vi "TDMS read for square (2).vi"() -> ()   [LabVIEW 2018]
uses:
  <vilib>/Analysis/Matrix/Numeric/Conversions/Array To Matrix - RA2.vi
  <vilib>/Analysis/Matrix/Numeric/Conversions/Matrix To Array - RM.vi
  <vilib>/Analysis/Matrix/NI_Matrix.lvlib
panel:
  out "result string":string
  out "string":string
  out "4":i32
  out "3":i32
  out "2":i32
  out "1":i32
  out "square X axis":dbl[][](graph)
  out "square Y axis":dbl[][](graph)
  in  "Scale:Multiplier":dbl=0.1
  in  "X Scale:Offset":dbl
  in  "Y Scale:Offset":dbl
  out "String":string
  in  "End Vector X":dbl
  in  "Start Vector X":dbl
  in  "End Vector Y":dbl
  in  "Start Vector Y":dbl
  out "Intensity Graph":dbl[][](graph)
  out "original X axis":dbl[][](graph)
  out "original Y axis":dbl[][](graph)
  in  "file path":path
  in  "OK Button":bool
  # "left side looking direction"
  # "right side looking direction"
  # "right side looking direction"
  # "left side looking direction"
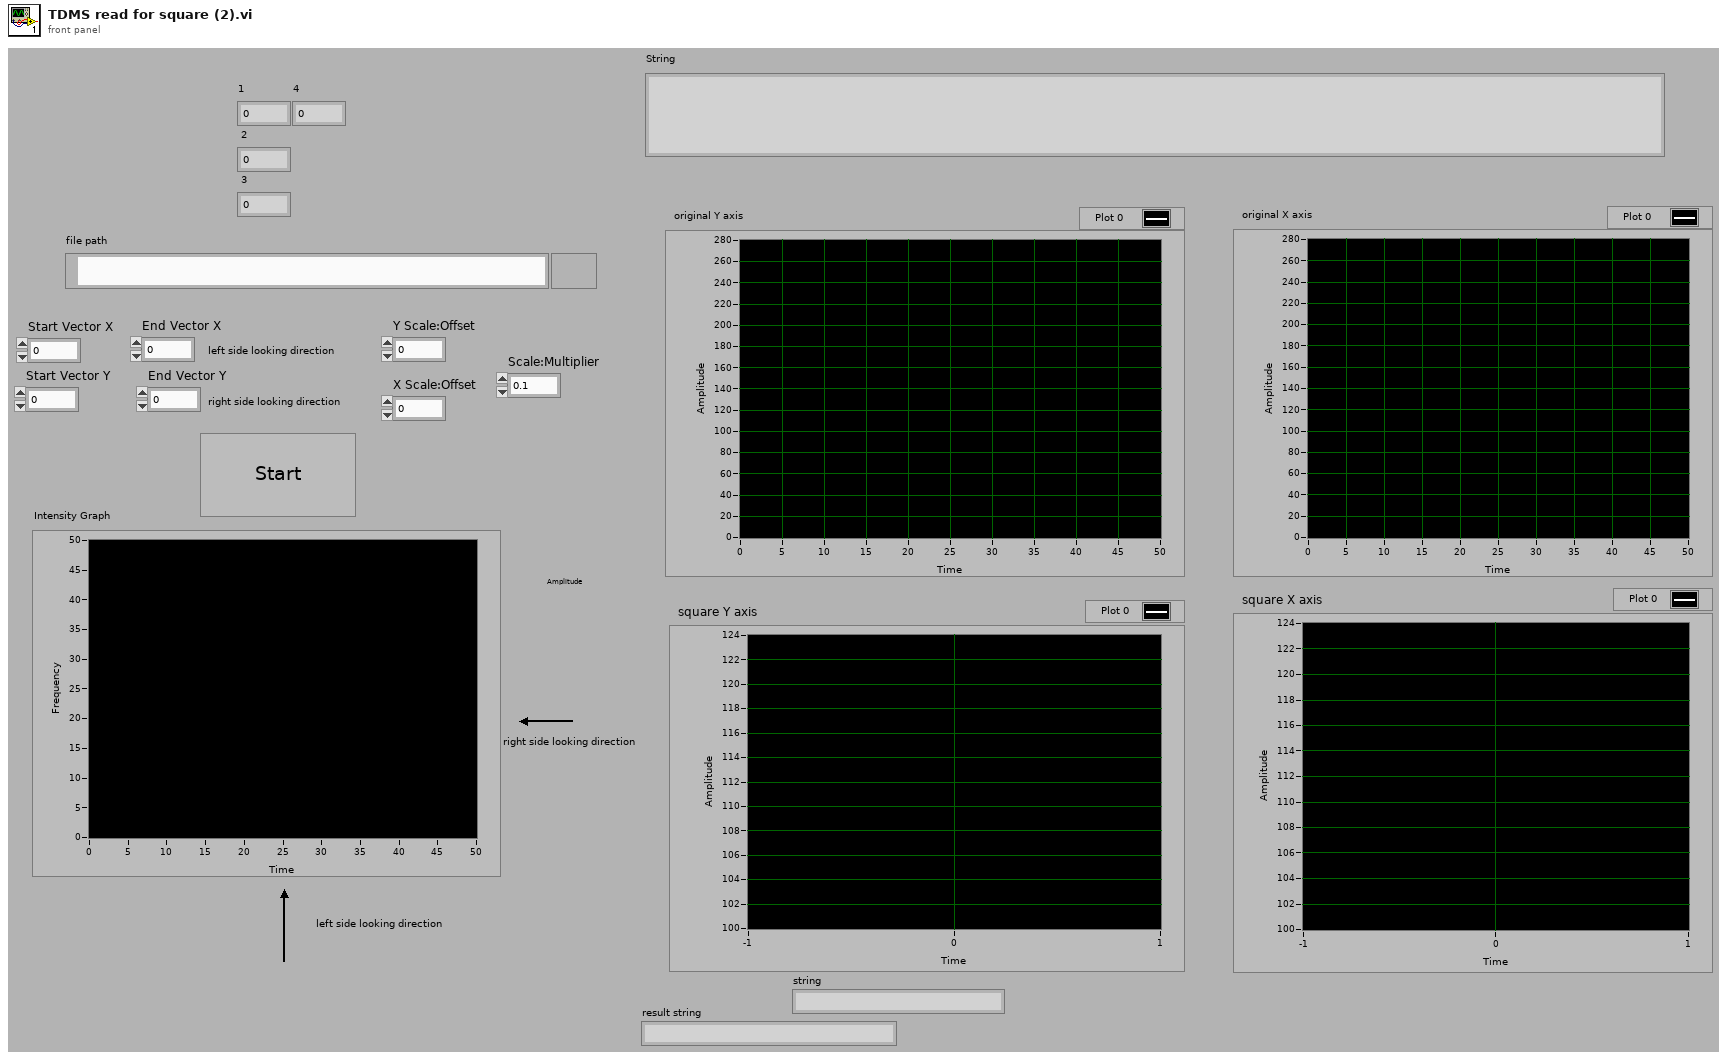
[diagram p1: front panel]
types:
  T1 = enum16{"open", "replace", "create", "open or create", "replace or create", "replace or create with confirmation"}
  T2 = enum16{"open", "open or create", "create or replace", "create", "open (read-only)"}
  T3 = typedef "NI_Matrix.lvlib/RealMatrix.ctl" = dbl[][]
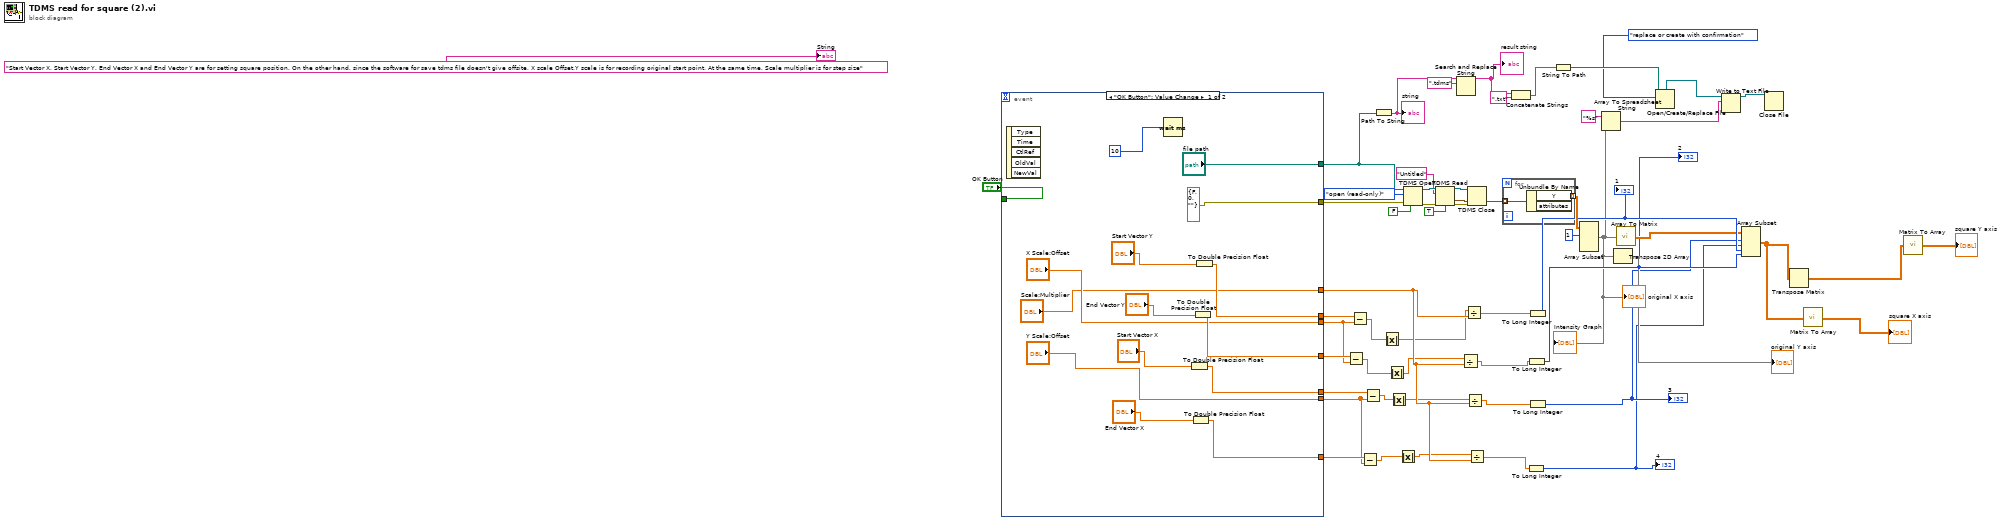
[diagram p0: block diagram]
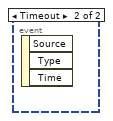
[diagram p2: hidden frame]
diagram:
  n1 = event shown="[0] \"OK Button\": Value Change" {
    selector: _ -> [_ _]
    dyn-events: _ -> [_ _]
    timeout: _ -> [_ _]
    tunnel: "OK Button" -> [_ _]
    tunnel: ["file path" _] -> w13
    tunnel: [errorcluster {"status"=FALSE, "code"=0, "source"=""} ("error constant") _] -> w46
    tunnel: [w66 _] -> w42
    tunnel: [w64 _] -> w41
    tunnel: [w61 _] -> w40
    tunnel: [w60 _] -> w39
    tunnel: ["X Scale:Offset" _] -> w38
    tunnel: ["Y Scale:Offset" _] -> w37
    tunnel: ["Scale:Multiplier" _] -> w36
    event "OK Button": Value Change {
      n2 = event-data() -> ()  [unwired: 1 in, 5 out]
      n3 = Wait (ms)(milliseconds to wait=u32 10) -> ()  [unwired: 1 out]
      n4 = To Double Precision Float(number="Start Vector X") -> (double precision float=w66:dbl)
      n5 = To Double Precision Float(number="End Vector X") -> (double precision float=w64:dbl)
      n6 = To Double Precision Float(number="End Vector Y") -> (double precision float=w60:dbl)
      n7 = To Double Precision Float(number="Start Vector Y") -> (double precision float=w61:dbl)
    }
    event Timeout {
      n8 = event-data() -> ()  [unwired: 1 in, 3 out]
    }
  }
  n9 = Subtract(x=w39, y=w38) -> (x-y=w29:dbl)
  n10 = Subtract(x=w40, y=w38) -> (x-y=w35:dbl)
  n11 = Subtract(x=w41, y=w37) -> (x-y=w33:dbl)
  n12 = Subtract(x=w42, y=w37) -> (x-y=w31:dbl)
  n13 = Path To String(path=w13) -> (string=w11:string)
  "string" <- w11
  n14 = Absolute Value(x=w35) -> (abs(x)=w34:dbl)
  n15 = Absolute Value(x=w29) -> (abs(x)=w28:dbl)
  n16 = Absolute Value(x=w31) -> (abs(x)=w30:dbl)
  n17 = Absolute Value(x=w33) -> (abs(x)=w32:dbl)
  n18 = TDMS Open(6:FALSE ("disable buffering? (T)"), 8:w46, 10:T2."open (read-only)" ("operation (0:open)"), 11:w13) -> (0:w51:errorcluster, 3:w53:refnum<k34>)  [unwired: 3 in]
  n19 = TDMS Read(0:w53, 5:"Untitled" ("group name in"), 11:w51, 13:TRUE ("return channels in file order? (F)")) -> (4:w52:refnum<k34>, 10:w49:waveform(dbl)[], 15:w50:errorcluster)  [unwired: 4 in, 3 out]
  n20 = Search and Replace String(input string=w11, search string=".tdms") -> (result string=w3:string)  [unwired: 6 in, 3 out]
  "result string" <- w3
  n21 = Divide(x=w28, y=w36) -> (x/y=w26:dbl)
  n22 = Divide(x=w34, y=w36) -> (x/y=w27:dbl)
  n23 = Divide(x=w30, y=w36) -> (x/y=w25:dbl)
  n24 = TDMS Close(8:w50, 11:w52) -> ()  [unwired: 2 out]
  n25 = Divide(x=w32, y=w36) -> (x/y=w24:dbl)
  n26 = for {
    tunnel: w49 -> [w72] mode=indexing
    tunnel: [w71] -> w45 mode=indexing
    n27 = Unbundle By Name(w72) -> ("Y"=w71:dbl[])  [unwired: 1 out]
  }
  n28 = Concatenate Strings(w3, ".txt" ("string")) -> (w1:string)
  n29 = To Long Integer(number=w24) -> (32bit integer=w18:i32)
  "4" <- w18
  n30 = To Long Integer(number=w26) -> (32bit integer=w20:i32)
  "2" <- w20
  n31 = To Long Integer(number=w25) -> (32bit integer=w19:i32)
  "3" <- w19
  n32 = To Long Integer(number=w27) -> (32bit integer=w22:i32)
  "1" <- w22
  n33 = String To Path(string=w1) -> (path=w9:path)
  n34 = Array Subset(array=w45, index (row)=1 ("index")) -> (w12:dbl[][])  [unwired: 3 in]
  "original X axis" <- w12
  "Intensity Graph" <- w12
  n35 = Array To Spreadsheet String(array=w12, 3:"%s" ("format string")) -> (spreadsheet string=w5:string)  [unwired: 1 in]
  n36 = Transpose 2D Array(2D array=w12) -> (transposed array=→"original Y axis":dbl[][])
  n37 = call-poly <vilib>:"Array To Matrix.vi"("Real 2D Array"=w12) -> ("Real Matrix"=w21:T3)
  n38 = Open/Create/Replace File(file path (use dialog)=w9, operation (0:open)=T1."replace or create with confirmation") -> (refnum out=w7:refnum<file>)  [unwired: 4 in, 2 out]
  n39 = Write to Text File(file (use dialog)=w7, text=w5) -> (refnum out=w4:refnum<file>)  [unwired: 2 in, 2 out]
  n40 = Array Subset(array=w21, index (row)=w19, length (row)=w18, index (col)=w22, length (col)=w20) -> (w17:T3)
  n41 = Close File(refnum=w4) -> ()  [unwired: 1 in, 2 out]
  n42 = Transpose Matrix(1:w17) -> (0:w16:T3)
  n43 = call-poly <vilib>:"Matrix To Array.vi"("Real Matrix"=w17) -> ("Real 2D Array"=→"square X axis":dbl[][])
  n44 = call-poly <vilib>:"Matrix To Array.vi"("Real Matrix"=w16) -> ("Real 2D Array"=→"square Y axis":dbl[][])
  "String" <- "Start Vector X, Start Vector Y, End Vector X and End Vector Y are for setting square position. On the other hand, since the software for save tdms file doesn't give offsite, X scale Offset,Y scale is for recording original start point. At the same time, Scale multiplier is for step size" ("String")
